vi "Is Bus Controller.vi"(8 "error in (no error)":errorcluster, 11 "1553 SubComponent":refnum<class "1553 SubComponent.lvclass">) -> (0 "error out":errorcluster)   [LabVIEW 2020, in "BCI-1553 API.lvlib" / "1553 Component.lvclass"]
doc: "Checks if the component is configured as a bus controller. A component that is configured as a bus controller will only have one Bus Controller subcomponent."
uses:
  1553 Component.lvclass
  1553 SubComponent/1553 SubComponent.lvclass
  Bus Controller/Bus Controller.lvclass
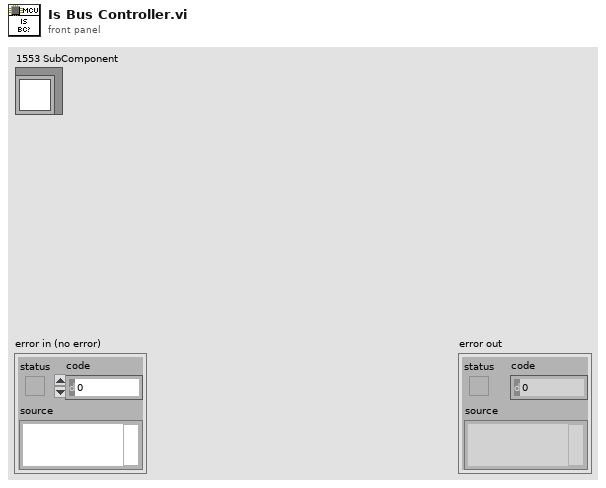
[diagram p1: front panel]
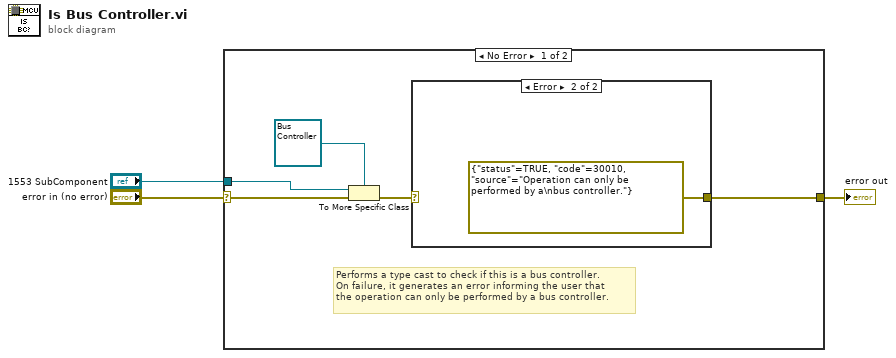
[diagram p0: block diagram]
diagram:
  n1 = case shown="No Error" "error in (no error)" {
    selector: "error in (no error)" -> [w7 w11]
    tunnel: [w4 w11] -> w2
    tunnel: "1553 SubComponent" -> [w8 _]
    frame No Error {
      # "Performs a type cast to check if this is a bus controller.\nOn failure, it generates an error informing the user that\nthe operation can only be performed by a bus controller."
      n2 = To More Specific Class(target class=refnum<class "Bus Controller.lvclass"> refnum ("SLSC 1553 API.lvlib:Bus Controller.lvclass"), reference=w8, error in=w7) -> (error out=w5:errorcluster)  [unwired: 1 out]
      n3 = case shown="Error" w5 {
        selector: w5 -> [w9 _]
        tunnel: [w9 errorcluster {"status"=TRUE, "code"=30010, "source"="Operation can only be performed by a\nbus controller."} ("error IO")] -> w4
        frame No Error {
        }
        frame Error {
        }
      }
    }
    frame Error {
    }
  }
  "error out" <- w2
